vi "Set LR Torque.vi"(6 "scaling":dbl=20.0 format="%#_13g", 8 "error in (no error)":errorcluster, 9 "FR RW":bool, 10 "Torque_Reference_HLR":dbl, 11 "TCP modebus instance in":refnum<class "Modbus Master.lvclass">[](array[class])) -> (0 "error out":errorcluster, 3 "TCP modebus instance out":refnum<class "Modbus Master.lvclass">[](array[class]))   [LabVIEW 2025]
uses:
  <vilib>/Modbus/master/Modbus Master.lvclass
  C:/Program Files/National Instruments/LabVIEW 2025/vi.lib/Modbus/subvis/Modbus API/Modbus API.lvclass
  <vilib>/Modbus/subvis/Modbus API/Modbus API.lvclass/Modbus API.ctl
  <vilib>/Modbus/subvis/Transmission Data Unit (ADU)/Transmission Data Unit/Transmission Data Unit.lvclass/Transmission Data Unit.ctl
  <vilib>/Modbus/master/Data Access/Unit ID/Set Unit ID Property.vi
  <vilib>/Modbus/subvis/Transmission Data Unit (ADU)/Transmission Data Unit/Data Access/Unit ID/Write Unit ID.vi
  <vilib>/Modbus/subvis/Modbus API/Read Transmission Data Unit.vi
  <vilib>/Modbus/subvis/Modbus API/Write Transmission Data Unit.vi
  <vilib>/Modbus/subvis/Transmission Data Unit (ADU)/Transmission Data Unit/Transmission Data Unit.lvclass
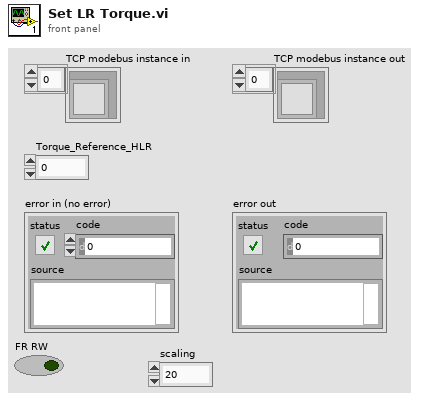
[diagram p1: front panel]
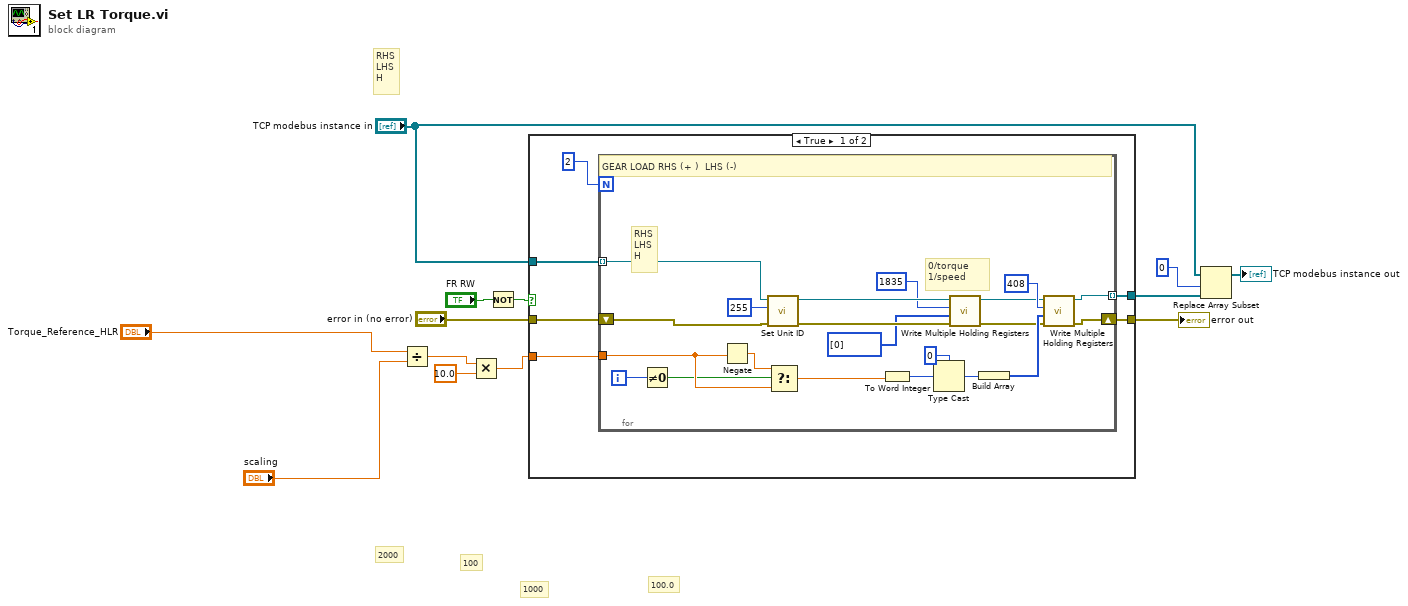
[diagram p0: block diagram]
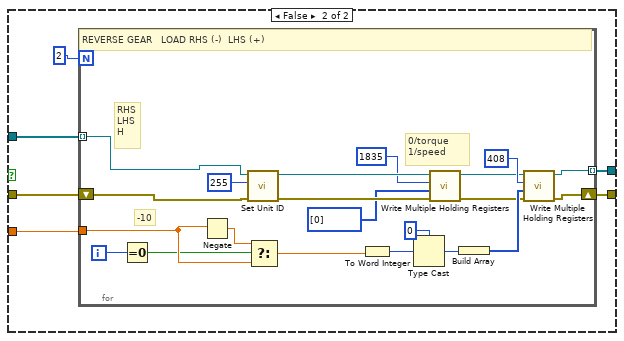
[diagram p2: hidden frame]
diagram:
  # "100.0"
  # "1000"
  # "100"
  # "2000"
  # "RHS\nLHS\nH"
  n1 = Divide(x="Torque_Reference_HLR", y="scaling") -> (x/y=w3:dbl)
  n2 = Multiply(x=w3, y=10.0) -> (x*y=w1:dbl)
  n3 = Not(x="FR RW") -> (.not. x?=w4:bool)
  n4 = case shown="True" w4 {
    tunnel: w1 -> [w19 w46]
    tunnel: [w18 w45] -> w11
    tunnel: "TCP modebus instance in" -> [w17 w44]
    tunnel: [w15 w42] -> w8
    tunnel: "error in (no error)" -> [w14 w41]
    frame True {
      n5 = for {
        N: 2 -> [_]
        tunnel: w19 -> [w22]
        shift-right: [w33] -> w15
        shift-left: w14 -> [w34]
        tunnel: w17 -> [w32] mode=indexing
        tunnel: [w31] -> w18 mode=indexing
        i -> [w30]
        # "RHS\nLHS\nH"
        # "0/torque\n1/speed"
        # "GEAR LOAD RHS (+ )  LHS (-)"
        n6 = Not Equal To 0?(x=w30) -> (x != 0?=w21:bool)
        n7 = Negate(x=w22) -> (-x=w20:dbl)
        n8 = call <vilib>:"Set Unit ID.vi"("error in (no error)"=w34, "unit ID"=u8 255, "Modbus master in"=w32) -> ("error out"=w28:errorcluster, "Modbus master out"=w26:refnum<class "Modbus Master.lvclass">)  [unwired: 7 in]
        n9 = Select(t=w20, s=w21, f=w22) -> (s? t:f=w29:dbl)
        n10 = To Word Integer(number=w29) -> (16bit integer=w38:i16)
        n11 = Type Cast(type=u16 0, x=w38) -> (*(type *) &x=w39:u16)
        n12 = call-dynamic "Write Multiple Holding Registers.vi"("error in (no error)"=w28, "holding register values"=u16[] [0], "starting address"=u16 1835, "Modbus master in"=w26) -> ("error out"=w27:errorcluster, "Modbus master out"=w25:refnum<class "Modbus Master.lvclass">)  [unwired: 6 in]
        n13 = Build Array(w39) -> (w35:u16[])
        n14 = call-dynamic "Write Multiple Holding Registers.vi"("error in (no error)"=w27, "holding register values"=w35, "starting address"=u16 408, "Modbus master in"=w25) -> ("error out"=w33:errorcluster, "Modbus master out"=w31:refnum<class "Modbus Master.lvclass">)  [unwired: 6 in]
      }
    }
    frame False {
      n15 = for {
        N: 2 -> [_]
        tunnel: w46 -> [w49]
        shift-right: [w60] -> w42
        shift-left: w41 -> [w61]
        tunnel: w44 -> [w59] mode=indexing
        tunnel: [w58] -> w45 mode=indexing
        i -> [w57]
        # "-10"
        # "RHS\nLHS\nH"
        # "0/torque\n1/speed"
        # "REVERSE GEAR   LOAD RHS (-)  LHS (+)"
        n16 = Equal To 0?(x=w57) -> (x = 0?=w48:bool)
        n17 = Negate(x=w49) -> (-x=w47:dbl)
        n18 = call <vilib>:"Set Unit ID.vi"("error in (no error)"=w61, "unit ID"=u8 255, "Modbus master in"=w59) -> ("error out"=w55:errorcluster, "Modbus master out"=w53:refnum<class "Modbus Master.lvclass">)  [unwired: 7 in]
        n19 = Select(t=w47, s=w48, f=w49) -> (s? t:f=w56:dbl)
        n20 = To Word Integer(number=w56) -> (16bit integer=w65:i16)
        n21 = Type Cast(type=u16 0, x=w65) -> (*(type *) &x=w66:u16)
        n22 = call-dynamic "Write Multiple Holding Registers.vi"("error in (no error)"=w55, "holding register values"=u16[] [0], "starting address"=u16 1835, "Modbus master in"=w53) -> ("error out"=w54:errorcluster, "Modbus master out"=w52:refnum<class "Modbus Master.lvclass">)  [unwired: 6 in]
        n23 = Build Array(w66) -> (w62:u16[])
        n24 = call-dynamic "Write Multiple Holding Registers.vi"("error in (no error)"=w54, "holding register values"=w62, "starting address"=u16 408, "Modbus master in"=w52) -> ("error out"=w60:errorcluster, "Modbus master out"=w58:refnum<class "Modbus Master.lvclass">)  [unwired: 6 in]
      }
    }
  }
  "error out" <- w8
  n25 = Replace Array Subset(array="TCP modebus instance in", new element=w11, index=0) -> (→"TCP modebus instance out":refnum<class "Modbus Master.lvclass">[])
